vi "Simple Occurrence.vi"() -> ()   [LabVIEW 2023]
doc: "Demonstrates how to continuously trigger the execution of a process from another process that runs in parallel, using Occurrences. Use the Occurrence functions to control separate, synchronous activities. In particular, use these functions when you want one part of a block diagram to wait until another part of a block diagram finishes a task.\n\nIn this example, two processes are running in parallel. An occurrence is generated by the Set Occurrence function in Loop 1 every time the current iteration is a multiple of 10. This occurrence is detected in Loop 2 by the Wait on Occurrence function."
uses:
  support/Global - Occurrence Loop Stop.vi
panel:
  out "Total Occurrences Fired":i32
  out "Current Loop 1 Iteration":i32
  in  "Stop":bool
  # "Overview: Demonstrates the use of the Occurrence functions to trigger the execution of a process from another process that runs in parallel.\nInstructions:\nRun the VI."
  # "On every tenth iteration of Loop 1, an occurrence will fire, causing Loop 2 to increment the Total Occurrences Fired count."
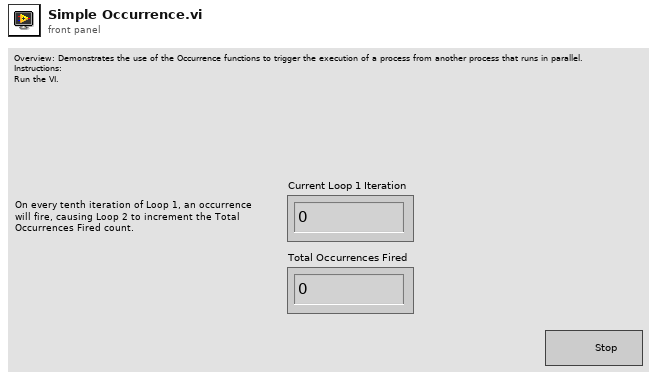
[diagram p1: front panel]
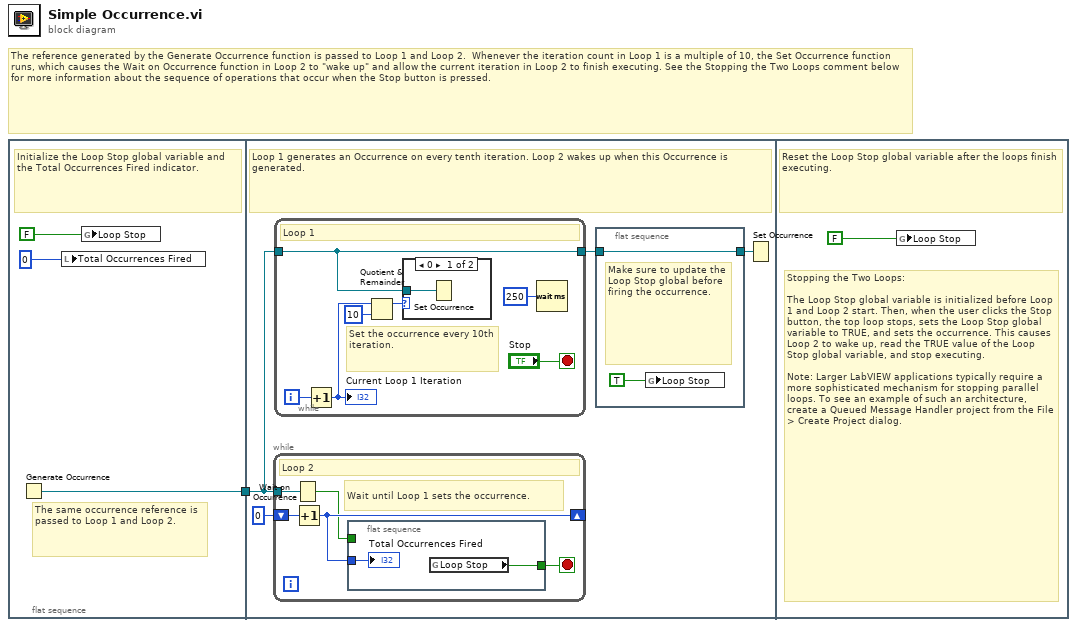
[diagram p0: block diagram]
diagram:
  # "The reference generated by the Generate Occurrence function is passed to Loop 1 and Loop 2.  Whenever the iteration count in Loop 1 is a multiple of 10, the Set Occurrence function runs, which causes the Wait on Occurrence function in Loop 2 to \"wake up\" and allow the current iteration in Loop 2 to finish executing. See the Stopping the Two Loops comment below for more information about the sequence of operations that occur when the Stop button is pressed."
  n1 = flat-sequence {
    tunnel: [w2] -> w1
    tunnel: w1 -> [w7]
    frame #0 {
      # "The same occurrence reference is passed to Loop 1 and Loop 2."
      # "Initialize the Loop Stop global variable and the Total Occurrences Fired indicator."
      n2 = Generate Occurrence() -> (w2:refnum<k4>)
      n3 = local write "Total Occurrences Fired"(0 ("Total Occurrences Fired")) -> ()
      n4 = global write "Global - Occurrence Loop Stop.vi" "Loop Stop"(FALSE ("Loop Stop")) -> ()
    }
    frame #1 {
      # "Loop 1 generates an Occurrence on every tenth iteration. Loop 2 wakes up when this Occurrence is generated."
      n5 = while {
        tunnel: w7 -> [w15]
        shift-right: [w13] -> _
        shift-left: 0 -> [w14]
        stop <- w12 stop-if-true
        # "Wait until Loop 1 sets the occurrence."
        # "Loop 2"
        n6 = Wait on Occurrence(2:w15) -> (0:w11:bool)  [unwired: 2 in]
        n7 = Increment(x=w14) -> (x+1=w13:i32)
        n8 = flat-sequence {
          tunnel: w13 -> [w17]
          tunnel: [w16] -> w12
          tunnel: w11 -> [_]
          frame #0 {
            n9 = global read "Global - Occurrence Loop Stop.vi" "Loop Stop"() -> (w16:bool)
            "Total Occurrences Fired" <- w17
          }
        }
      }
      n10 = while {
        tunnel: w7 -> [w20]
        tunnel: [w20] -> w6
        i -> [w24]
        stop <- "Stop" stop-if-true
        # "Set the occurrence every 10th iteration."
        # "Loop 1"
        n11 = Increment(x=w24) -> (x+1=w23:i32)
        "Current Loop 1 Iteration" <- w23
        n12 = Quotient & Remainder(x=w23, y=10) -> (x-y*floor(x/y)=w21:i32)  [unwired: 1 out]
        n13 = case shown="0" w21 {
          tunnel: w20 -> [w25 _]
          frame 0 {
            n14 = Set Occurrence(w25) -> ()
          }
          frame Default {
          }
        }
        n15 = Wait (ms)(milliseconds to wait=u32 250) -> ()  [unwired: 1 out]
      }
      n16 = flat-sequence {
        tunnel: [w10] -> w5
        tunnel: w6 -> [w10]
        frame #0 {
          # "Make sure to update the Loop Stop global before firing the occurrence."
          n17 = global write "Global - Occurrence Loop Stop.vi" "Loop Stop"(TRUE ("Loop Stop")) -> ()
        }
      }
      n18 = Set Occurrence(w5) -> ()
    }
    frame #2 {
      # "Stopping the Two Loops:\n\nThe Loop Stop global variable is initialized before Loop 1 and Loop 2 start. Then, when the user clicks the Stop button, the top loop stops, sets the Loop Stop global variable to TRUE, and sets the occurrence. This causes Loop 2 to wake up, read the TRUE value of the Loop Stop global variable, and stop executing.\n\nNote: Larger LabVIEW applications typically require a more sophisticated mechanism for stopping parallel loops. To see an example of such an architecture, create a Queued Message Handler project from the File > Create Project dialog."
      # "Reset the Loop Stop global variable after the loops finish executing."
      n19 = global write "Global - Occurrence Loop Stop.vi" "Loop Stop"(FALSE ("Loop Stop")) -> ()
    }
  }
